vi "Write Remove View Timeout (1000 ms).vi"(8 "error in (no error)":errorcluster, 10 "Remove View Timeout (1000 ms)":i32=1000, 11 "GUI View Actor in":refnum<class "GUI View Actor.lvclass">) -> (0 "error out":errorcluster, 3 "GUI View Actor out":refnum<class "GUI View Actor.lvclass">)   [LabVIEW 2017, in "GUI Views.lvlib" / "GUI View Actor.lvclass"]
uses:
  GUI View Actor.lvclass
  GUI View Actor.lvclass/GUI View Actor.ctl
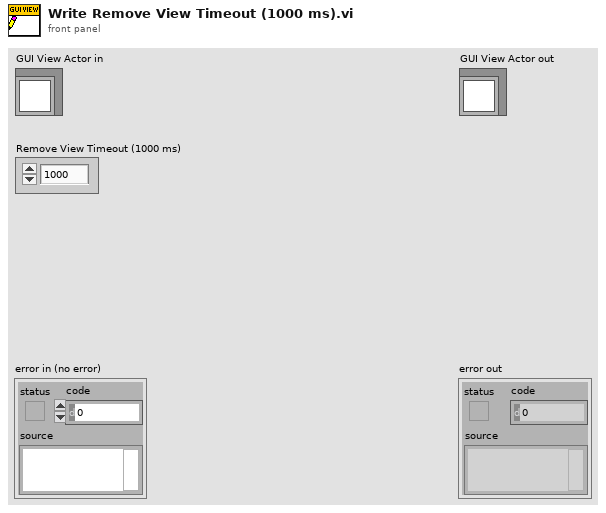
[diagram p1: front panel]
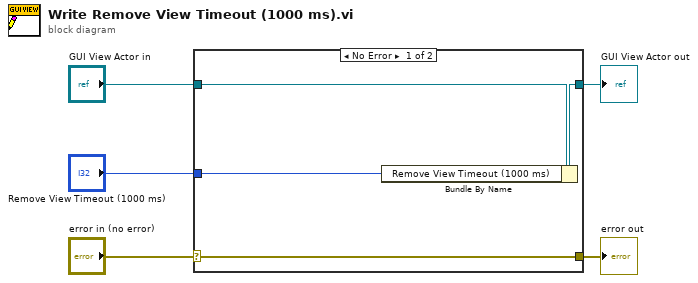
[diagram p0: block diagram]
diagram:
  n1 = case shown="No Error" "error in (no error)" {
    selector: "error in (no error)" -> [w9 w10]
    tunnel: [w9 w10] -> w4
    tunnel: [w7 w11] -> w2
    tunnel: "GUI View Actor in" -> [w8 w11]
    tunnel: "Remove View Timeout (1000 ms)" -> [w6 _]
    frame No Error {
      n2 = Bundle By Name(cluster=w8, "Remove View Timeout (1000 ms)"=w6) -> (w7:refnum<class "GUI View Actor.lvclass">)
    }
    frame Error {
    }
  }
  "error out" <- w4
  "GUI View Actor out" <- w2
